vi "TCPIP_CRLF_Quary.vi"(3 "错误输入（无错误）":errorcluster, 4 "指令":string, 5 "连接ID":refnum<k5>) -> (0 "错误输出":errorcluster, 1 "数据输出":string, 2 "连接ID输出":refnum<k5>)   [LabVIEW 2018]
panel:
  # "CRLF 指令后需要加入\\r\\n"
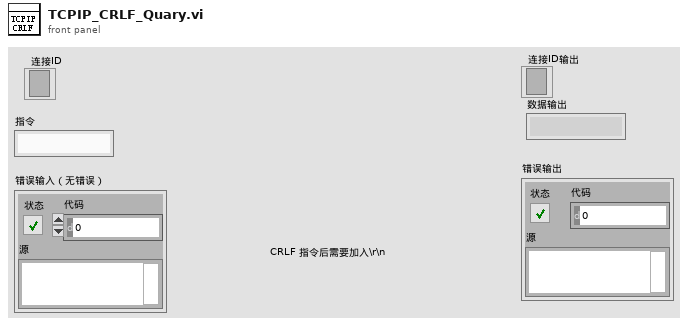
[diagram p1: front panel]
types:
  T1 = enum16{"Standard", "Buffered", "CRLF", "Immediate"}
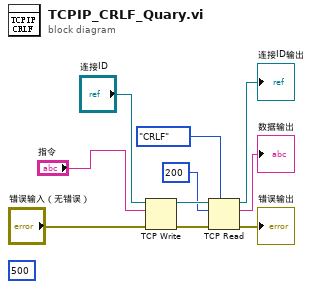
[diagram p0: block diagram]
diagram:
  (unwired) 500 ("读取的字节")
  n1 = TCP Write(connection ID="连接ID", data in="指令", error in (no error)="错误输入（无错误）") -> (connection ID out=w6:refnum<k5>, error out=w9:errorcluster)  [unwired: 1 in, 1 out]
  n2 = TCP Read(connection ID=w6, bytes to read=200 ("读取的字节"), error in (no error)=w9, 7:T1."CRLF" ("模式（标准）")) -> (connection ID out=→"连接ID输出":refnum<k5>, data out=→"数据输出":string, error out=→"错误输出":errorcluster)  [unwired: 1 in]
